vi "Door_02.vi"(7 "Mode":T2(ring), 8 "error in (no error)":errorcluster, 11 "Queue In":T1) -> (0 "error out":errorcluster, 3 "Queue Out":T1)   [LabVIEW 2011]
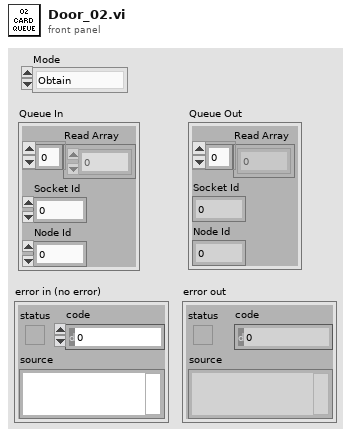
[diagram p1: front panel]
types:
  T1 = cluster{"Read Array":u8[], "Socket Id":u8, "Node Id":u8}
  T2 = enum16{"Obtain", "Enqueue", "Dequeue", "Release"}
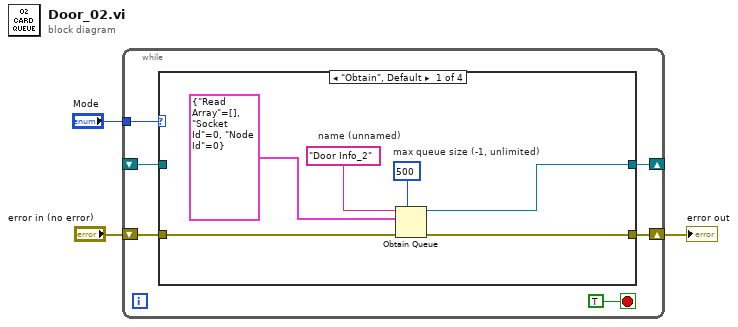
[diagram p0: block diagram]
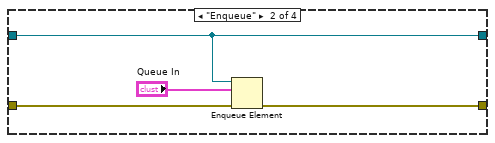
[diagram p2: hidden frame]
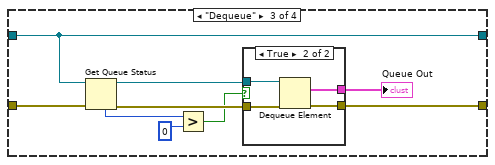
[diagram p3: hidden frame]
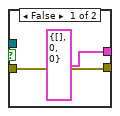
[diagram p4: hidden frame]
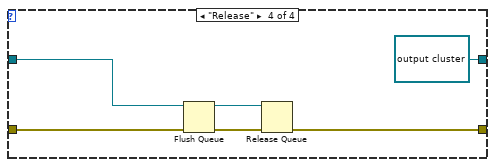
[diagram p5: hidden frame]
diagram:
  n1 = while {
    tunnel: "Mode" -> [w9]
    shift-right: [w7] -> w1
    shift-left: "error in (no error)" -> [w8]
    shift-right: [w6] -> _
    shift-left: _ -> [w5]
    stop <- TRUE stop-if-true
    n2 = case shown="\"Obtain\", Default" w9 {
      tunnel: w8 -> [w15 w19 w27 w39]
      tunnel: [w14 w18 w28 w38] -> w7
      tunnel: [w12 w17 w25 refnum<queue> refnum ("queue out")] -> w6
      tunnel: w5 -> [_ w17 w25 w37]
      frame "Obtain", Default {
        w11 = 500  # max queue size (-1, unlimited)
        w13 = "Door Info_2"  # name (unnamed)
        n3 = Obtain Queue(max queue size (-1, unlimited)=w11, name (unnamed)=w13, element data type=T1 {"Read Array"=[], "Socket Id"=0, "Node Id"=0} ("output cluster"), error in (no error)=w15) -> (queue out=w12:refnum<queue>, error out=w14:errorcluster)  [unwired: 1 in, 1 out]
      }
      frame "Enqueue" {
        n4 = Enqueue Element(queue=w17, element="Queue In", error in (no error)=w19) -> (error out=w18:errorcluster)  [unwired: 1 in, 2 out]
      }
      frame "Dequeue" {
        n5 = Get Queue Status(queue=w25, error in (no error)=w27) -> (queue out=w24:refnum<queue>, error out=w26:errorcluster, # elements in queue=w22:i32)  [unwired: 1 in, 5 out]
        n6 = Greater?(x=w22, y=0) -> (0:w21:bool)
        n7 = case shown="True" w21 {
          tunnel: [w30 w34] -> w28
          tunnel: [T1 {"Read Array"=[], "Socket Id"=0, "Node Id"=0} ("output cluster") w33] -> w20
          tunnel: w26 -> [w30 w32]
          tunnel: w24 -> [_ w31]
          frame False {
          }
          frame True {
            n8 = Dequeue Element(queue=w31, error in (no error)=w32) -> (element=w33:T1, error out=w34:errorcluster)  [unwired: 1 in, 2 out]
          }
        }
        "Queue Out" <- w20
      }
      frame "Release" {
        n9 = Flush Queue(queue=w37) -> (queue out=w35:refnum<queue>)  [unwired: 1 in, 2 out]
        n10 = Release Queue(queue=w35, error in (no error)=w39) -> (error out=w38:errorcluster)  [unwired: 1 in, 2 out]
      }
    }
  }
  "error out" <- w1
